vi "Calc XY (SubVI)_v1.vi"(10 "Grid Settings":T1, 11 "element":i64) -> (0 "y2":dbl, 1 "x2":dbl, 2 "y_i":i64, 3 "x_i":i64)   [LabVIEW 2014]
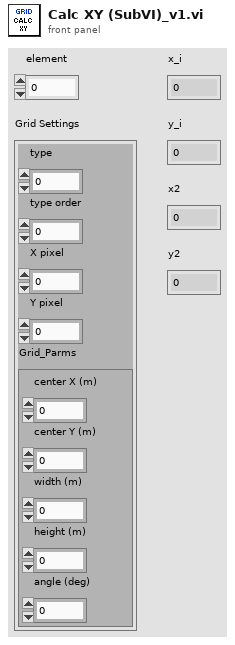
[diagram p1: front panel]
types:
  T1 = cluster{"type":u16, "type order":u16, "X pixel":dbl, "Y pixel":dbl, "Grid_Parms":cluster{"center X (m)":sgl, "center Y (m)":sgl, "width (m)":sgl, "height (m)":sgl, "angle (deg)":sgl}}
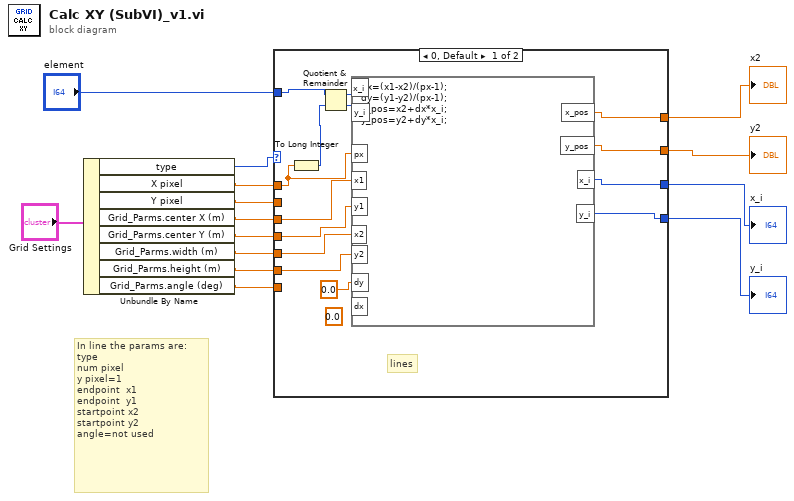
[diagram p0: block diagram]
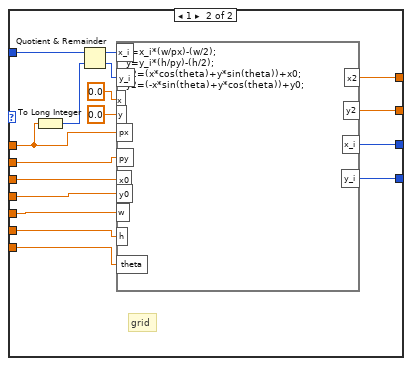
[diagram p2: hidden frame]
diagram:
  # "In line the params are:\ntype\nnum pixel\ny pixel=1\nendpoint  x1\nendpoint  y1\nstartpoint x2\nstartpoint y2\nangle=not used"
  n1 = Unbundle By Name("Grid Settings") -> ("type"=w1:u16, "X pixel"=w5:dbl, "Y pixel"=w6:dbl, "Grid_Parms.center X (m)"=w7:sgl, "Grid_Parms.center Y (m)"=w8:sgl, "Grid_Parms.width (m)"=w2:sgl, "Grid_Parms.height (m)"=w3:sgl, "Grid_Parms.angle (deg)"=w4:sgl)
  n2 = case shown="0, Default" w1 {
    tunnel: [w16 w45] -> w14
    tunnel: [w17 w44] -> w13
    tunnel: [w27 w41] -> w11
    tunnel: [w28 w40] -> w10
    tunnel: "element" -> [w25 w38]
    tunnel: w8 -> [w21 w37]
    tunnel: w7 -> [w22 w36]
    tunnel: w6 -> [_ w35]
    tunnel: w5 -> [w18 w34]
    tunnel: w4 -> [_ w33]
    tunnel: w3 -> [w19 w32]
    tunnel: w2 -> [w20 w31]
    frame 0, Default {
      (unwired) sgl 0.0 ("output variable")
      # "lines"
      n3 = To Long Integer(number=w18) -> (32bit integer=w26:i32)
      n4 = Quotient & Remainder(x=w25, y=w26) -> (x-y*floor(x/y)=w24:i64, floor(x/y)=w23:i64)
      n5 = formula code="dx=(x1-x2)/(px-1);\ndy=(y1-y2)/(px-1);\nx_pos=x2+dx*x_i;\ny_pos=y2+dy*x_i;"("x_i"=w24, "y_i"=w23, "y2"=w19, "x2"=w20, "px"=w18, "x1"=w22, "y1"=w21, "dy"=0.0 ("input variable")) -> ("x_pos"=w17:dbl, "y_pos"=w16:dbl, "x_i"=w28:i64, "y_i"=w27:i64)  [unwired: 1 out]
    }
    frame 1 {
      # "grid"
      n6 = To Long Integer(number=w34) -> (32bit integer=w30:i32)
      n7 = Quotient & Remainder(x=w38, y=w30) -> (x-y*floor(x/y)=w39:i64, floor(x/y)=w29:i64)
      n8 = formula code="x=x_i*(w/px)-(w/2);\ny=y_i*(h/py)-(h/2);\nx2=(x*cos(theta)+y*sin(theta))+x0;\ny2=(-x*sin(theta)+y*cos(theta))+y0;"("x_i"=w39, "y_i"=w29, "w"=w31, "h"=w32, "theta"=w33, "py"=w35, "px"=w34, "x0"=w36, "y0"=w37, "x"=0.0 ("input variable"), "y"=0.0 ("input variable")) -> ("x2"=w44:dbl, "y2"=w45:dbl, "x_i"=w40:i64, "y_i"=w41:i64)
    }
  }
  "y2" <- w14
  "x2" <- w13
  "y_i" <- w11
  "x_i" <- w10
